vi "CameraSync.vi"(11 "IO Cluster In":T1={"Error"={"status"=FALSE, "code"=0, "source"=""}, "Encoder Calibration Values"=[22, 216], "Update Calibration"=FALSE, "JPEG Resolutions"=3, "Raw Resolutions"=1, "Image Mode"=enum."RAW Gray Scale", "FPGA Ref"=refnum} {"JPEG Resolutions" items=["160x128"=3, "320x240"=5, "640x480"=7]; "Raw Resolutions" items=["80x60"=1, "160x120"=3, "128x128"=9, "128x96"=11]}) -> (1 "Max Attempts Reached":bool, 2 "Sync Complete":bool, 3 "IO Cluster Out":T1={"Error"={"status"=FALSE, "code"=0, "source"=""}, "Encoder Calibration Values"=[22, 216], "Update Calibration"=FALSE, "JPEG Resolutions"=3, "Raw Resolutions"=1, "Image Mode"=enum."RAW Gray Scale", "FPGA Ref"=refnum} {"JPEG Resolutions" items=["160x128"=3, "320x240"=5, "640x480"=7]; "Raw Resolutions" items=["80x60"=1, "160x120"=3, "128x128"=9, "128x96"=11]})   [LabVIEW 2019]
uses:
  QNET MS IO Cluster.ctl
panel:
  out "Attempt":i32
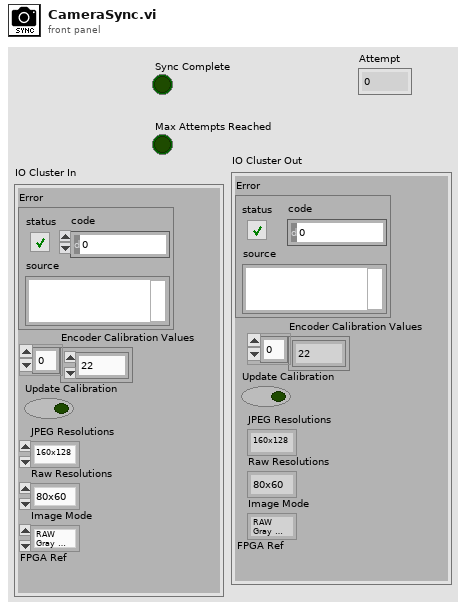
[diagram p1: front panel]
types:
  T1 = typedef "QNET MS IO Cluster.ctl" = cluster{"Error":errorcluster, "Encoder Calibration Values":i32[], "Update Calibration":bool, "JPEG Resolutions":u16, "Raw Resolutions":u16, "Image Mode":enum16{"RAW RGB", "RAW Gray Scale", "JPEG"}, "FPGA Ref":refnum<k20>}
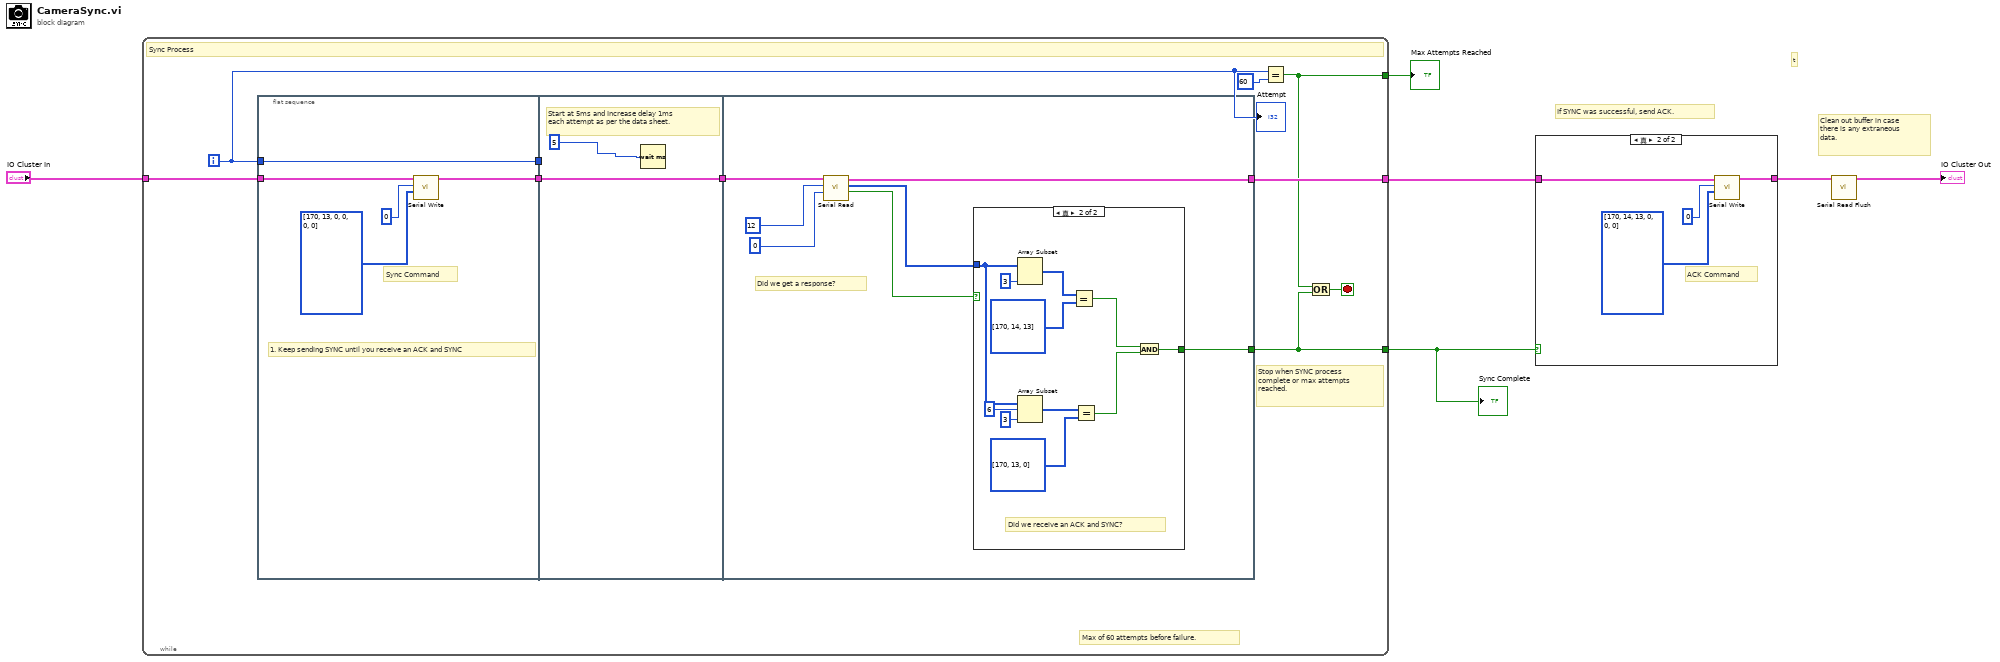
[diagram p0: block diagram]
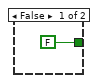
[diagram p3: hidden frame]
diagram:
  # "t"
  # "Clean out buffer in case\nthere is any extraneous\ndata."
  # "If SYNC was successful, send ACK."
  n1 = while {
    tunnel: "IO Cluster In" -> [w16]
    tunnel: [w7] -> w6
    tunnel: [w9] -> w5
    tunnel: [w8] -> w3
    i -> [w15]
    stop <- w13 stop-if-true
    # "Stop when SYNC process\ncomplete or max attempts \nreached."
    # "Max of 60 attempts before failure."
    # "Sync Process"
    n2 = flat-sequence {
      tunnel: w16 -> [w19]
      tunnel: [w18] -> w12
      tunnel: w15 -> [w17]
      tunnel: [w17] -> w11
      tunnel: w12 -> [w23]
      tunnel: w11 -> [_]
      tunnel: [w23] -> w10
      tunnel: w10 -> [w26]
      tunnel: [w25] -> w9
      tunnel: [w24] -> w8
      frame #0 {
        # "1. Keep sending SYNC until you receive an ACK and SYNC"
        # "Sync Command"
        n3 = call "Serial Write.vi"("Array"=u8[] [170, 13, 0, 0, 0, 0], "Timeout (ms)"=0, "IO Cluster In"=w19) -> ("IO Cluster Out"=w18:T1)  [unwired: 8 in]
      }
      frame #1 {
        # "Start at 5ms and Increase delay 1ms \neach attempt as per the data sheet."
        n4 = Wait (ms)(milliseconds to wait=u32 5) -> ()  [unwired: 1 out]
      }
      frame #2 {
        # "Did we get a response?"
        n5 = call "Serial Read.vi"("Timeout (ms)"=0, "Number of Bytes to Read"=u32 12 ("Number of Elements"), "IO Cluster In"=w26) -> ("Data Valid"=w29:bool, "Data"=w30:u8[], "IO Cluster Out"=w25:T1)  [unwired: 4 in, 2 out]
        n6 = case shown="真" w29 {
          tunnel: w30 -> [_ w38]
          tunnel: [FALSE w32] -> w24
          frame False {
          }
          frame True {
            # "Did we receive an ACK and SYNC?"
            n7 = Array Subset(array=w38, length=3) -> (w41:u8[])  [unwired: 1 in]
            n8 = Array Subset(array=w38, index=6, length=3) -> (w36:u8[])
            n9 = Equal?(x=w41, y=u8[] [170, 14, 13]) -> (x = y?=w34:bool)
            n10 = Equal?(x=w36, y=u8[] [170, 13, 0]) -> (x = y?=w33:bool)
            n11 = And(x=w34, y=w33) -> (x .and. y?=w32:bool)
          }
        }
      }
    }
    n12 = Equal?(x=w15, y=60) -> (x = y?=w7:bool)
    n13 = Or(x=w7, y=w8) -> (x .or. y?=w13:bool)
    "Attempt" <- w15
  }
  "Max Attempts Reached" <- w6
  "Sync Complete" <- w3
  n14 = case shown="真" w3 {
    tunnel: w5 -> [w43 w45]
    tunnel: [w43 w44] -> w4
    frame False {
    }
    frame True {
      # "ACK Command"
      n15 = call "Serial Write.vi"("Array"=u8[] [170, 14, 13, 0, 0, 0], "Timeout (ms)"=0, "IO Cluster In"=w45) -> ("IO Cluster Out"=w44:T1)  [unwired: 8 in]
    }
  }
  n16 = call "Serial Read Flush.vi"("IO Cluster In"=w4) -> ("IO Cluster Out"=→"IO Cluster Out":T1)  [unwired: 10 in]
